vi "values checker.vi"(8 "error in (no error)":errorcluster, 9 "values 1":string[](array[string]), 10 "values 2":string[](array[string]), 11 "sections":string[][](array[string])) -> (0 "error out":errorcluster)   [LabVIEW 2024]
doc: "<b>values 1</b> stores the current selections of the ring controls, structured as follows: [name1,index1,name2,index2,name3,index3,...]\nEach name represents the selected item in a ring control, and the corresponding index indicates its position in the control’s list.\n\n<b>values 2</b> contains the full list of possible items for all ring controls, structured as follows: [name1_ctrl1, name2_ctrl1, name3_ctrl1, ...,\n name1_ctrl2, name2_ctrl2, name3_ctrl2, ..., name1_ctrl3, name2_ctrl3, name3_ctrl3, ...]\n\nNOTE: Each ring control has a predefined number of items, and this determines its maximum index.\n\n<b>sections</b> only provides the number of keys in each section, where each section represents a Ring control.\n\nThis VI performs two validation checks:\n1.- Ensures that every selected name in <b>values 1</b> exists within <b>values 2</b>.\n2.- Confirms that each index in <b>values 1</b> does not exceed the maximum allowed for its corresponding control in <b>values 2</b>."
uses:
  <vilib>/Utility/error.llb/Error Cluster From Error Code.vi
  <vilib>/ErrorRing/Error Ring.xnode
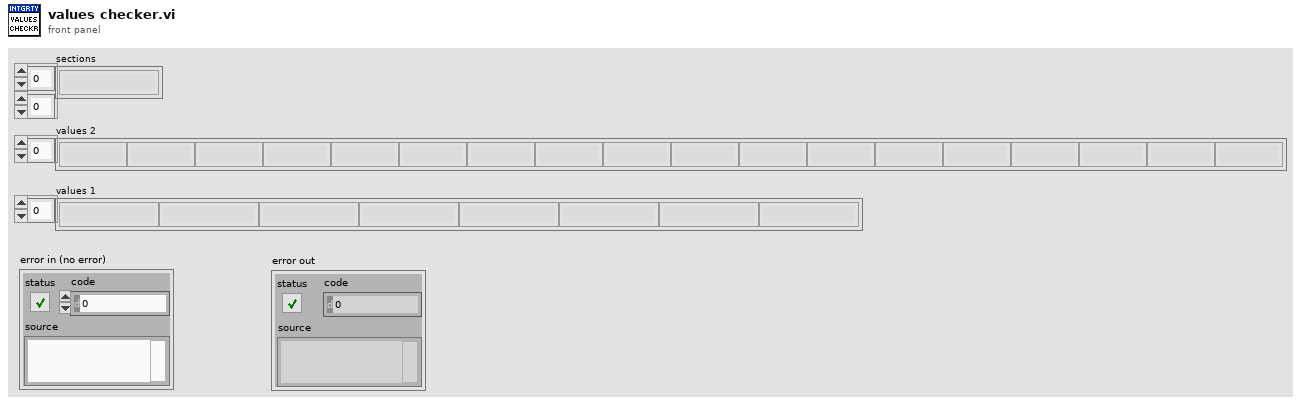
[diagram p1: front panel]
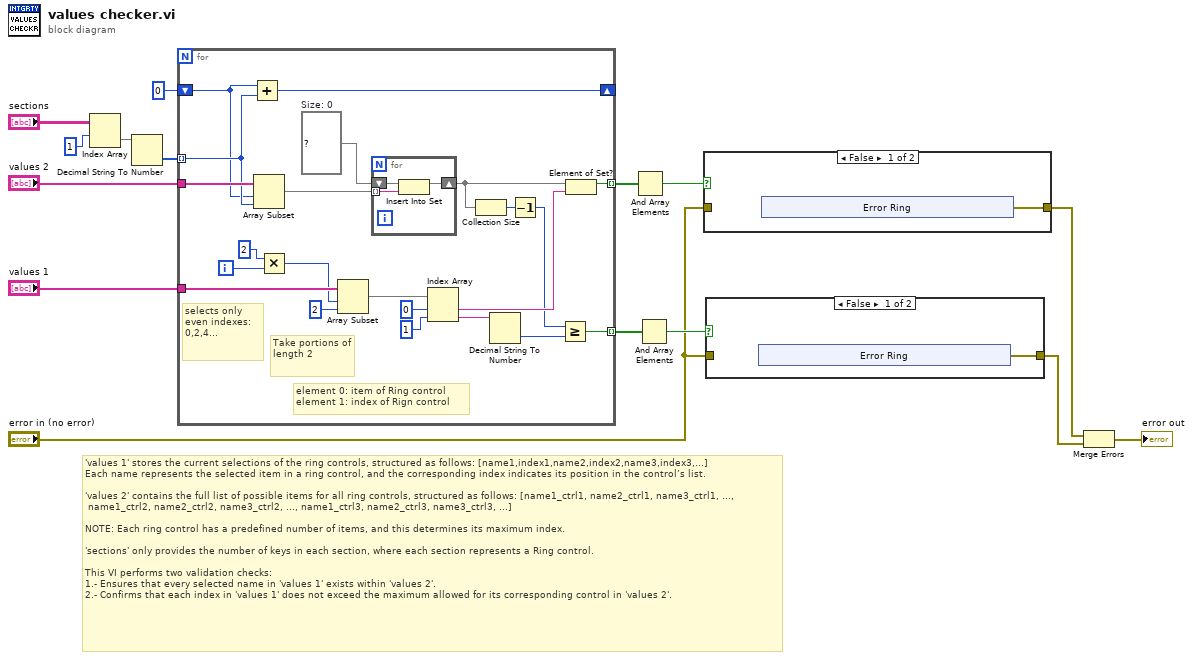
[diagram p0: block diagram]
diagram:
  # "'values 1' stores the current selections of the ring controls, structured as follows: [name1,index1,name2,index2,name3,index3,...]\nEach name represents the selected item in a ring control, and the corresponding index indicates its position in the control’s list.\n\n'values 2' contains the full list of possible items for all ring controls, structured as follows: [name1_ctrl1, name2_ctrl1, name3_ctrl1, ...,\n name1_ctrl2, name2_ctrl2, name3_ctrl2, ..., name1_ctrl3, name2_ctrl3, name3_ctrl3, ...]\n\nNOTE: Each ring control has a predefined number of items, and this determines its maximum index.\n\n'sections' only provides the number of keys in each section, where each section represents a Ring control.\n\nThis VI performs two validation checks:\n1.- Ensures that every selected name in 'values 1' exists within 'values 2'.\n2.- Confirms that each index in 'values 1' does not exceed the maximum allowed for its corresponding control in 'values 2'."
  n1 = Index Array(array="sections", index (row)=1) -> (element=w11:string[])  [unwired: 1 in]
  n2 = Decimal String To Number(string=w11) -> (number=w14:i32[])  [unwired: 2 in, 1 out]
  n3 = for {
    tunnel: w14 -> [w34] mode=indexing
    shift-right: [w37] -> _
    shift-left: 0 -> [w33]
    tunnel: "values 2" -> [w36]
    tunnel: "values 1" -> [w35]
    tunnel: [w18] -> w8 mode=indexing
    tunnel: [w17] -> w7 mode=indexing
    i -> [w31]
    w27 = set{string} {}  # Size: 0
    # "element 0: item of Ring control\nelement 1: index of Rign control"
    # "Take portions of length 2"
    # "selects only even indexes: 0,2,4..."
    n4 = Add(x=w33, y=w34) -> (x+y=w37:i32)
    n5 = Array Subset(array=w36, index=w33, length=w34) -> (w28:string[])
    n6 = Multiply(x=2, y=w31) -> (x*y=w29:i32)
    n7 = Array Subset "Array Subset"(array=w35, index=w29, length=2) -> (w26:string[])
    n8 = for {
      tunnel: w28 -> [w40] mode=indexing
      shift-right: [w38] -> w23
      shift-left: w27 -> [w39]
      n9 = Insert Into Set(10:w40, 11:w39) -> (3:w38:set{string})  [unwired: 1 out]
    }
    n10 = Index Array "Index Array"(array=w26, index #1=0 ("index"), index #2=1 ("index")) -> (element #1=w22:string, element #2=w21:string)
    n11 = Collection Size(1:w23) -> (0:w20:i32)
    n12 = Decimal String To Number(string=w21) -> (number=w19:i32)  [unwired: 2 in, 1 out]
    n13 = Decrement(x=w20) -> (x-1=w16:i32)
    n14 = Greater Or Equal?(x=w16, y=w19) -> (x >= y?=w17:bool)
    n15 = Element of Set?(10:w22, 11:w23) -> (3:w18:bool)
  }
  n16 = And Array Elements(Boolean array=w8) -> (logical AND=w5:bool)
  n17 = And Array Elements(Boolean array=w7) -> (logical AND=w6:bool)
  n18 = case shown="False" w5 {
    tunnel: [w41 w47] -> w1
    tunnel: "error in (no error)" -> [_ w47]
    frame False {
      n19 = xnode ("Error Ring")() -> ("error out"=w41:errorcluster)
    }
    frame True {
    }
  }
  n20 = case shown="False" w6 {
    tunnel: [w48 w54] -> w2
    tunnel: "error in (no error)" -> [_ w54]
    frame False {
      n21 = xnode ("Error Ring")() -> ("error out"=w48:errorcluster)
    }
    frame True {
    }
  }
  n22 = Merge Errors(w1, w2) -> (→"error out":errorcluster)
